vi "Remove Zero Coefficients (DBL).vi"(9 "threshold type":T1 items=["Absolute Value", "Relative Value"], 10 "threshold":dbl, 11 "P(x) In":dbl[](array[numeric]) format="%#.6g") -> (0 "error":i32, 2 "number of zero coefficients":i32, 3 "P(x) Out":dbl[](array[numeric]) format="%#.6g")   [LabVIEW 2019, in "NI_AALPro.lvlib"]
doc: "Removes from <B>P(x) In</B> the trailing coefficients near zero whose absolute values are less than <B>threshold</B>. Wire data to the <B>P(x) In</B> input to determine the polymorphic instance to use or manually select the instance."
uses:
  NI_AALPro.lvlib
  Remove Zero Threshold Type.ctl
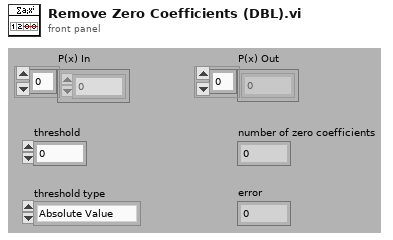
[diagram p1: front panel]
types:
  T1 = typedef "NI_AALPro.lvlib/Remove Zero Threshold Type.ctl" = u16
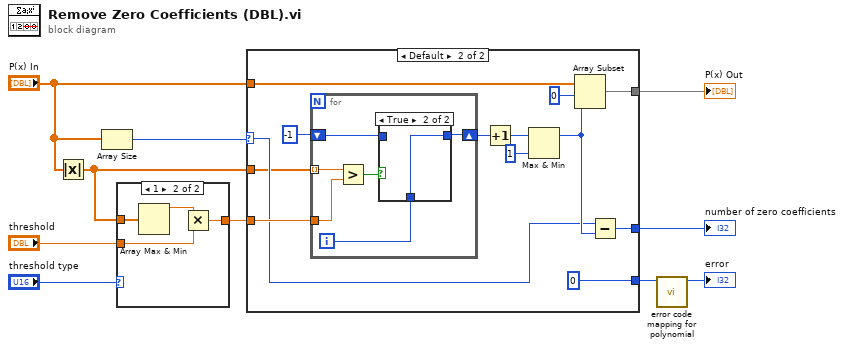
[diagram p0: block diagram]
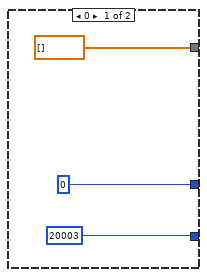
[diagram p3: hidden frame]
diagram:
  n1 = Absolute Value(x="P(x) In") -> (abs(x)=w1:dbl[])
  n2 = Array Size(array="P(x) In") -> (size(s)=w9:i32)
  n3 = case shown="1" "threshold type" {
    tunnel: "threshold" -> [w11 w13]
    tunnel: [w11 w12] -> w2
    tunnel: w1 -> [_ w15]
    frame 0, Default {
    }
    frame 1 {
      n4 = Array Max & Min(array=w15) -> (max value=w14:dbl)  [unwired: 3 out]
      n5 = Multiply(x=w14, y=w13) -> (x*y=w12:dbl)
    }
  }
  n6 = case shown="Default" w9 {
    selector: w9 -> [_ w21]
    tunnel: [dbl[] [] ("BDL") w26] -> w10
    tunnel: "P(x) In" -> [_ w25]
    tunnel: w2 -> [_ w24]
    tunnel: [20003 ("empty array") 0] -> w7
    tunnel: [0 w20] -> w8
    tunnel: w1 -> [_ w19]
    frame 0 {
    }
    frame Default {
      n7 = for {
        shift-right: [w36] -> w30
        shift-left: -1 -> [w35]
        tunnel: w24 -> [w34]
        tunnel: w19 -> [w32] mode=indexing
        i -> [w37]
        n8 = Greater?(x=w32, y=w34) -> (0:w33:bool)
        n9 = case shown="True" w33 {
          tunnel: w37 -> [_ w39]
          tunnel: [w38 w39] -> w36
          tunnel: w35 -> [w38 _]
          frame False {
          }
          frame True {
          }
        }
      }
      n10 = Increment(x=w30) -> (x+1=w28:i32)
      n11 = Max & Min(x=w28, y=1) -> (max(x,y)=w22:i32)  [unwired: 1 out]
      n12 = Array Subset(array=w25, index=0, length=w22) -> (w26:dbl[])
      n13 = Subtract(x=w21, y=w22) -> (x-y=w20:i32)
    }
  }
  "P(x) Out" <- w10
  "number of zero coefficients" <- w8
  n14 = call "error code mapping for polynomial.vi"("error in"=w7) -> ("error out"=→"error":i32)  [unwired: 10 in]
